vi "Controller.vi"(0 "UART_Command":T2, 5 "Cmd_data":u16, 7 "RX":bool) -> (4 "UART_Reply":T1, 6 "Reply_data":u16, 8 "TX":bool, 10 "TX_Busy":bool, 14 "Rate (Ticks)":u32 caption="Tick Count (ticks)", 15 "RX_Busy":bool)   [LabVIEW 2015, in "UART_Firmware.lvlib"]
uses:
  UART_Firmware.lvlib
  UART_Command.ctl
  UART_Response.ctl
  Settings.ctl
  Parity.ctl
  StopBits.ctl
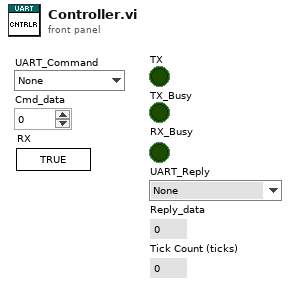
[diagram p1: front panel]
types:
  T1 = typedef "UART_Firmware.lvlib/UART_Response.ctl" = enum8{"None", "Rx", "BaudHighAck", "BaudLowAck", "CharSizeAck", "ParityAck", "StopBitsAck", "SpacingHighAck", "SpacingLowAck", "ParityError", "FrameError"}
  T2 = typedef "UART_Firmware.lvlib/UART_Command.ctl" = enum8{"None", "Tx", "SetBaud_High", "SetBaud_Low", "SetCharLength", "SetParity", "SetStopBits", "SetSpacing_High", "SetSpacing_Low"}
  T3 = typedef "UART_Firmware.lvlib/Settings.ctl" = cluster{"Baud (ticks)":u32, "CharacterSize":u8, "Parity":T4, "Stop Bits":T5, "Spacing (ticks)":u32}
  T4 = typedef "UART_Firmware.lvlib/Parity.ctl" = enum8{"None", "Even", "Odd"}
  T5 = typedef "UART_Firmware.lvlib/StopBits.ctl" = enum8{"1.0", "1.5", "2.0"}
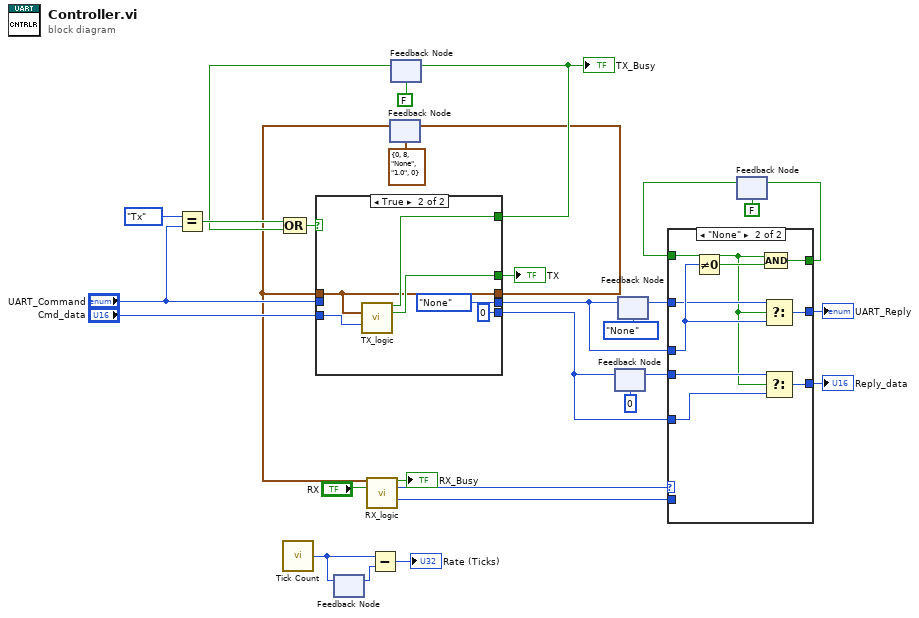
[diagram p0: block diagram]
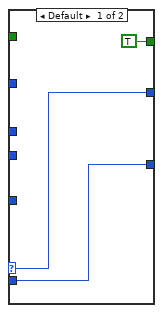
[diagram p2: hidden frame]
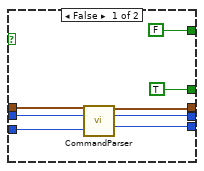
[diagram p3: hidden frame]
diagram:
  n1 = Equal?(x=UART_Command."Tx" ("y"), y="UART_Command") -> (x = y?=w30:bool)
  n2 = call "Tick Count"() -> ("Tick Count(Ticks)"=w11:u32)
  n3 = feedback-in #1(w11) -> ()
  n4 = feedback #1() -> (w12:u32)  [unwired: 1 in]
  n5 = Subtract(x=w11, y=w12) -> (x-y=→"Rate (Ticks)":u32)
  n6 = feedback #2(T3 {"Baud (ticks)"=0, "CharacterSize"=8, "Parity"=enum."None", "Stop Bits"=enum."1.0", "Spacing (ticks)"=0} ("Settings")) -> (w2:T3)
  n7 = call "RX_logic.vi"("Settings"=w2, "Rx"="RX") -> ("Busy"=→"RX_Busy":bool, "RX_reply"=w9:T1, "Rx_data"=w19:u16)  [unwired: 10 in, 1 out]
  n8 = feedback #3(FALSE ("Busy")) -> (w20:bool)
  n9 = Compound Arithmetic op=OR(w30, w20) -> (w29:bool)
  n10 = case shown="True" w29 {
    tunnel: [TRUE ("TX") w44] -> w28
    tunnel: [FALSE ("Busy") w43] -> w22
    tunnel: "UART_Command" -> [w35 _]
    tunnel: "Cmd_data" -> [w34 w42]
    tunnel: [w36 w39] -> w1
    tunnel: [w33 UART_Response."None" ("UART Reply")] -> w25
    tunnel: [w32 u16 0 ("Reply_Data")] -> w17
    tunnel: w2 -> [w31 w39]
    frame False {
      n11 = call "CommandParser.vi"("Settings in"=w31, "UART_Command"=w35, "Cmd_data"=w34) -> ("Settings out"=w36:T3, "UART Reply"=w33:T1, "Reply_Data"=w32:u16)  [unwired: 10 in]
    }
    frame True {
      n12 = call "TX_logic.vi"("Settings"=w39, "TX_data"=w42) -> ("Busy"=w43:bool, "TX"=w44:bool)  [unwired: 12 in]
    }
  }
  "TX" <- w28
  "TX_Busy" <- w22
  n13 = feedback-in #2(w1) -> ()
  n14 = feedback-in #3(w22) -> ()
  n15 = feedback #4(u16 0 ("Reply_Data")) -> (w15:u16)
  n16 = feedback-in #4(w17) -> ()
  n17 = feedback #5(UART_Response."None" ("UART Reply")) -> (w26:T1)
  n18 = feedback-in #5(w25) -> ()
  n19 = feedback #6(FALSE) -> (w6:bool)
  n20 = case shown="\"None\"" w9 {
    selector: w9 -> [w46 _]
    tunnel: w26 -> [_ w53]
    tunnel: w25 -> [_ w54]
    tunnel: w19 -> [w47 _]
    tunnel: w17 -> [_ w51]
    tunnel: [w47 w55] -> w13
    tunnel: w15 -> [_ w52]
    tunnel: [w46 w56] -> w14
    tunnel: [TRUE w49] -> w8
    tunnel: w6 -> [_ w48]
    frame Default {
    }
    frame "None" {
      n21 = Not Equal To 0?(x=w54) -> (x != 0?=w50:bool)
      n22 = Select(t=w53, s=w48, f=w54) -> (s? t:f=w56:T1)
      n23 = Select(t=w52, s=w48, f=w51) -> (s? t:f=w55:u16)
      n24 = Compound Arithmetic op=AND(w48, w50) -> (w49:bool)
    }
  }
  "UART_Reply" <- w14
  "Reply_data" <- w13
  n25 = feedback-in #6(w8) -> ()
